vi "Should Swap.vi"(9 "Person B":T1={"ID"=0, "Family Name"="Doe", "Given Name"="John", "Birth Date"=timestamp(3533142714.9178333 s since 1904-01-01)} {"Birth Date" format="%<%Y/%b/%d>T"}, 10 "Person A":T1={"ID"=0, "Family Name"="Smith", "Given Name"="John", "Birth Date"=timestamp(3533056306.0488334 s since 1904-01-01)} {"Birth Date" format="%<%Y/%b/%d>T"}, 11 "Swapper Using Given Name in":refnum<class "Swapper Using Year Born.lvclass">) -> (2 "Swap?":bool)   [LabVIEW 2023, in "Swapper Using Year Born.lvclass"]
uses:
  Swapper Using Year Born.lvclass
  Person Information.ctl
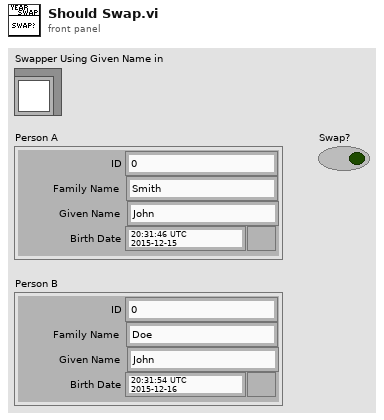
[diagram p1: front panel]
types:
  T1 = typedef "Person Information.ctl" = cluster{"ID":u32, "Family Name":string, "Given Name":string, "Birth Date":timestamp}
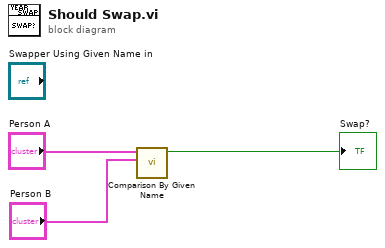
[diagram p0: block diagram]
diagram:
  n1 = call "Comparison By Given Name.vi"("Person B"="Person B", "Person A"="Person A") -> ("Swap?"=→"Swap?":bool)  [unwired: 9 in]
